vi "RPC Method PerformACIRMeasurement.vi"(8 "error in (no error)":errorcluster, 11 "OOP Server in":refnum<class "OCV3.lvclass">) -> (0 "error out":errorcluster, 3 "OOP Server out":refnum<class "OCV3.lvclass">)   [LabVIEW 2019, in "OCV3.lvlib" / "OCV3.lvclass"]
uses:
  OCV3.lvclass
  OCV3.lvclass/OCV3.ctl
  RPC Messages/measurementservice_ErrorOut/measurementservice_ErrorOut_Data.ctl
  RPC Messages/measurementservice_ACIRRaw/measurementservice_ACIRRaw_Data.ctl
  RPC Messages/measurementservice_ACIRData/measurementservice_ACIRData_Data.ctl
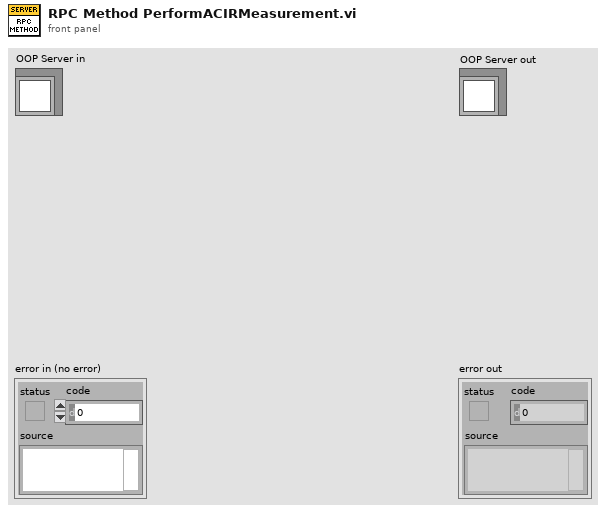
[diagram p1: front panel]
types:
  T1 = typedef "OCV3.lvlib/OCV3.lvclass/measurementservice_ErrorOut_Data.ctl" = cluster{"errCode":i32, "errMessage":string}
  T2 = typedef "OCV3.lvlib/OCV3.lvclass/measurementservice_ACIRRaw_Data.ctl" = cluster{"Impedance":sgl, "Real":sgl, "Imaginery":sgl, "error":T1}
  T3 = typedef "OCV3.lvlib/OCV3.lvclass/measurementservice_ACIRData_Data.ctl" = cluster{"data":T2[]}
  T4 = typedef "OCV3.lvlib/OCV3.lvclass/Server Internal UEs.ctl" = cluster{"Invoke Internal UE":refnum<user-event>, "Query Internal UE":refnum<user-event>, "PerformOCVMeasurement Internal UE":refnum<user-event>, "PerformACIRMeasurement Internal UE":refnum<user-event>, "StreamOCVMeasurement Internal UE":refnum<user-event>, "Register Internal UE":refnum<user-event>}
  T5 = typedef "OCV3.lvlib/OCV3.lvclass/Server gRPC UEs.ctl" = cluster{"Invoke gRPC UE":refnum<user-event>, "Query gRPC UE":refnum<user-event>, "PerformOCVMeasurement gRPC UE":refnum<user-event>, "PerformACIRMeasurement gRPC UE":refnum<user-event>, "StreamOCVMeasurement gRPC UE":refnum<user-event>, "Register gRPC UE":refnum<user-event>}
  T6 = typedef "OCV3.lvlib/gprc-lvsupport.lvlib/grpcId.ctl" = u64
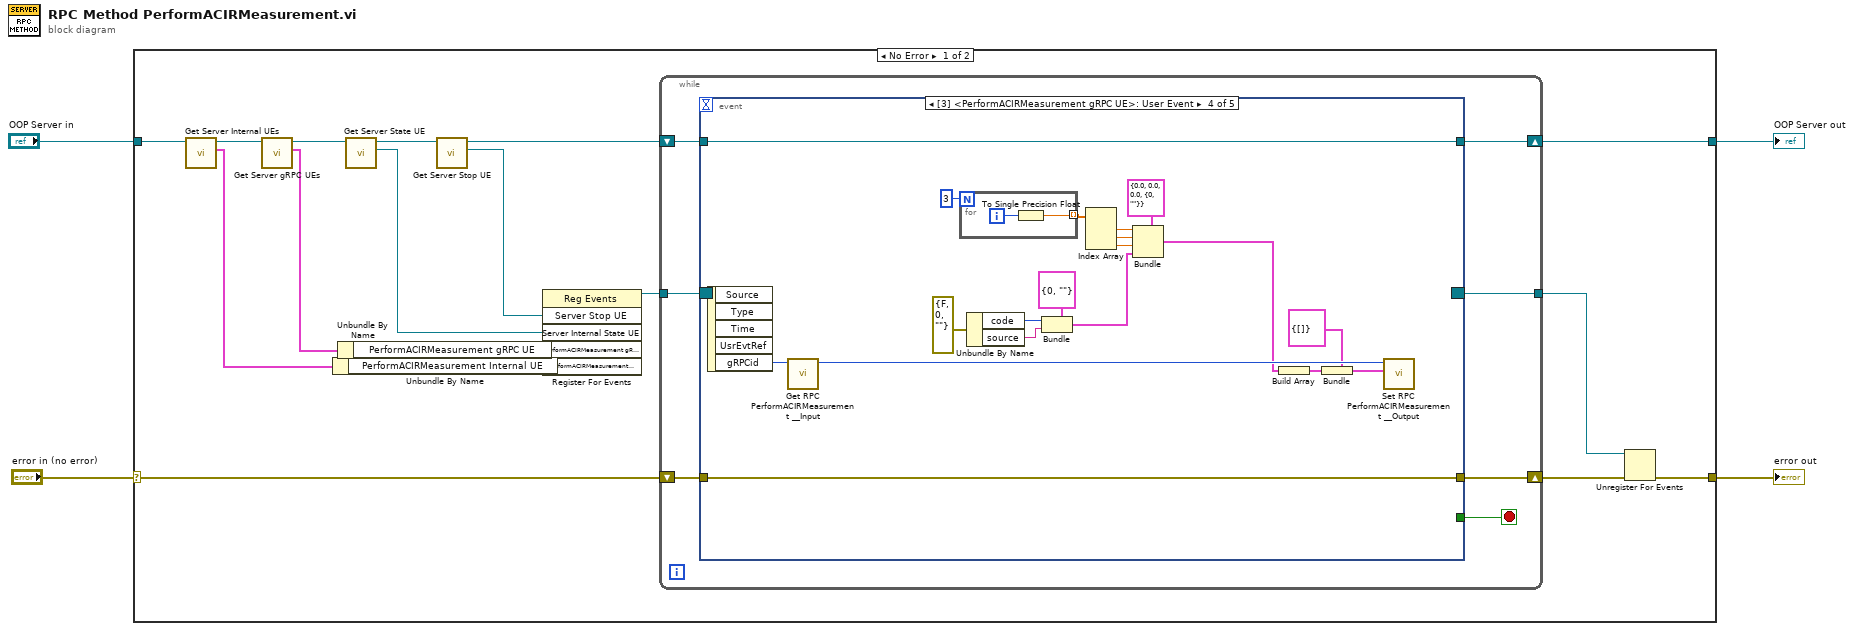
[diagram p0: block diagram]
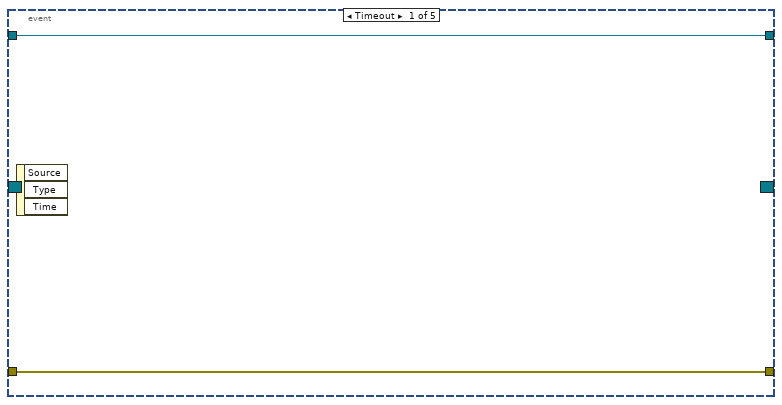
[diagram p2: hidden frame]
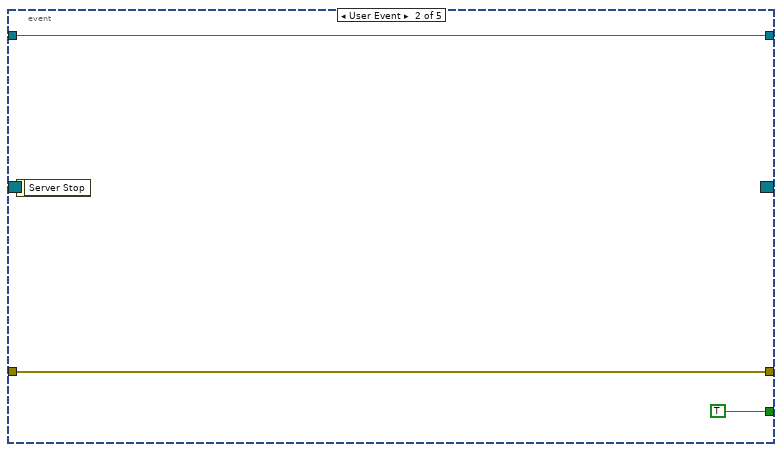
[diagram p3: hidden frame]
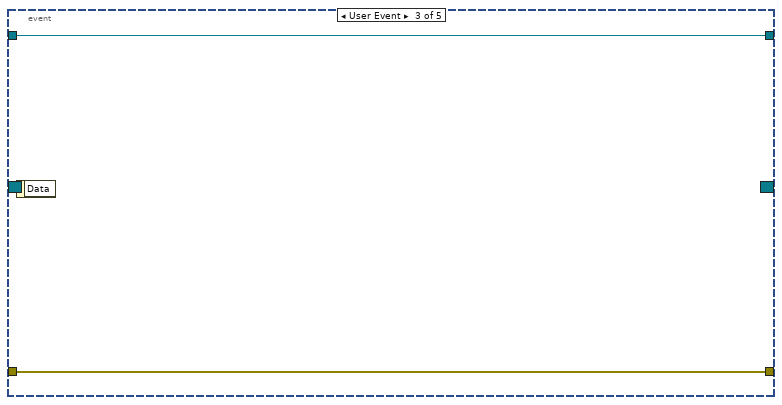
[diagram p4: hidden frame]
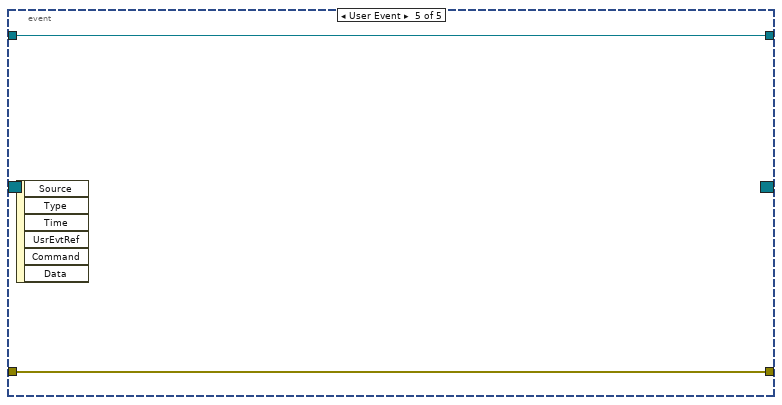
[diagram p5: hidden frame]
diagram:
  n1 = case shown="No Error" "error in (no error)" {
    selector: "error in (no error)" -> [w17 w60]
    tunnel: [w15 w60] -> w3
    tunnel: "OOP Server in" -> [w19 w59]
    tunnel: [w5 w59] -> w1
    frame No Error {
      n2 = call "Get Server Internal UEs.vi"("OOP Server in"=w19) -> ("Server Internal UEs"=w11:T4, "OOP Server out"=w18:refnum<class "OCV3.lvclass">)  [unwired: 9 in]
      n3 = call "Get Server gRPC UEs.vi"("OOP Server in"=w18) -> ("Server gRPC UEs"=w13:T5, "OOP Server out"=w8:refnum<class "OCV3.lvclass">)  [unwired: 9 in]
      n4 = Unbundle By Name ("Unbundle Internal UE")(w11) -> ("PerformACIRMeasurement Internal UE"=w10:refnum<user-event>)
      n5 = Unbundle By Name ("Unbundle gRPC UE")(w13) -> ("PerformACIRMeasurement gRPC UE"=w12:refnum<user-event>)
      n6 = call "Get Server State UE.vi"("Template Server in"=w8) -> ("Server Internal State UE"=w6:refnum<user-event>, "Template Server out"=w7:refnum<class "OCV3.lvclass">)  [unwired: 9 in]
      n7 = call "Get Server Stop UE.vi"("OOP Server in"=w7) -> ("Server Stop UE"=w21:refnum<user-event>, "OOP Server out"=w9:refnum<class "OCV3.lvclass">)  [unwired: 9 in]
      n8 = register-events(w21, w6, w12, w10) -> (reference out=w20:refnum<event-registration>)  [unwired: 2 in, 1 out]
      n9 = while {
        tunnel: w20 -> [w28]
        tunnel: [w24] -> w14
        shift-right: [w25] -> w16
        shift-left: w17 -> [w26]
        shift-right: [w22] -> w5
        shift-left: w9 -> [w23]
        stop <- w27 stop-if-true
        n10 = event "RPC Method Event Structure" shown="[3] <PerformACIRMeasurement gRPC UE>: User Event" {
          selector: w28 -> [_ _ _ _ _]
          dyn-events: [_ _ _ _ _] -> w24
          timeout: _ -> [_ _ _ _ _]
          tunnel: [_ TRUE _ _ _] -> w27
          tunnel: w26 -> [w30 w32 w35 w54 w58]
          tunnel: [w30 w32 w35 w54 w58] -> w25
          tunnel: w23 -> [w29 w31 w34 w53 w57]
          tunnel: [w29 w31 w34 w53 w57] -> w22
          event Timeout {
            n11 = event-data() -> ()  [unwired: 1 in, 3 out]
          }
          event User Event {
            n12 = event-data() -> ()  [unwired: 1 in, 1 out]
          }
          event User Event {
            n13 = event-data() -> ()  [unwired: 1 in, 1 out]
          }
          event User Event {
            n14 = event-data() -> ("gRPCid"=w50:T6)  [unwired: 1 in, 4 out]
            n15 = call "Get RPC PerformACIRMeasurement __Input.vi"("gRPCid in"=w50) -> ("gRPCid out"=w49:T6)  [unwired: 8 in, 2 out]
            n16 = for {
              N: 3 -> [_]
              tunnel: [w56] -> w39 mode=indexing
              i -> [w55]
              n17 = To Single Precision Float(number=w55) -> (single precision float=w56:sgl)
            }
            n18 = Unbundle By Name(errorcluster {"status"=FALSE, "code"=0, "source"=""} ("error in (no error)")) -> ("code"=w42:i32, "source"=w41:string)
            n19 = Bundle(cluster=T1 {"errCode"=0, "errMessage"=""} ("measurementservice_ErrorOut_Data"), "errCode"=w42, "errMessage"=w41) -> (w40:T1)
            n20 = Index Array(array=w39) -> (element #1=w38:sgl, element #2=w37:sgl, element #3=w36:sgl)  [unwired: 3 in]
            n21 = Bundle(cluster=T2 {"Impedance"=0.0, "Real"=0.0, "Imaginery"=0.0, "error"={"errCode"=0, "errMessage"=""}} ("measurementservice_ACIRRaw_Data"), "Impedance"=w38, "Real"=w37, "Imaginery"=w36, "error"=w40) -> (w44:T2)
            n22 = Build Array(w44) -> (w45:T2[])
            n23 = Bundle(cluster=T3 {"data"=[]} ("Message Data"), "data"=w45) -> (w47:T3)
            n24 = call "Set RPC PerformACIRMeasurement __Output.vi"("Message Data"=w47, "gRPCid in"=w49) -> ()  [unwired: 9 in, 1 out]
          }
          event User Event {
            n25 = event-data() -> ()  [unwired: 1 in, 6 out]
          }
        }
      }
      n26 = Unregister For Events(event registration refnum=w14, error in=w16) -> (error out=w15:errorcluster)
    }
    frame Error {
    }
  }
  "error out" <- w3
  "OOP Server out" <- w1
